vi "Emulator_VI_template.vi"() -> ()   [LabVIEW 2020]
uses:
  <vilib>/Instr/_visa.llb/VISA Configure Serial Port (Instr).vi
panel:
  in  "Start":bool
  in  "Stop":bool
  in  "Serial port configuration":T1={"Baud rate"=0, "Data bits"=5, "Parity"=enum."None", "Stop bits"=0, "Flow control"=0} {"Flow control" items=["None"=0, "XON/XOFF"=1, "RTS/CTS"=2, "DTR/DSR"=4]; "Stop bits" items=["1.0"=10, "1.5"=15, "2.0"=20]; "Data bits" min=5 max=8 step=1; "Baud rate" items=["9600"=9600, "19200"=19200, "38400"=38400, "57600"=57600, "115200"=115200]}
  in  "Port":refnum<visa-resource-name>
  # "Project name:  Emulator_VI_template.vi \nDescription:     Template VI for emulation interface communicating with external target through UART port\nVersion:           01.00\nRevision:          00\nLast modified : MM/DD/YYYY"
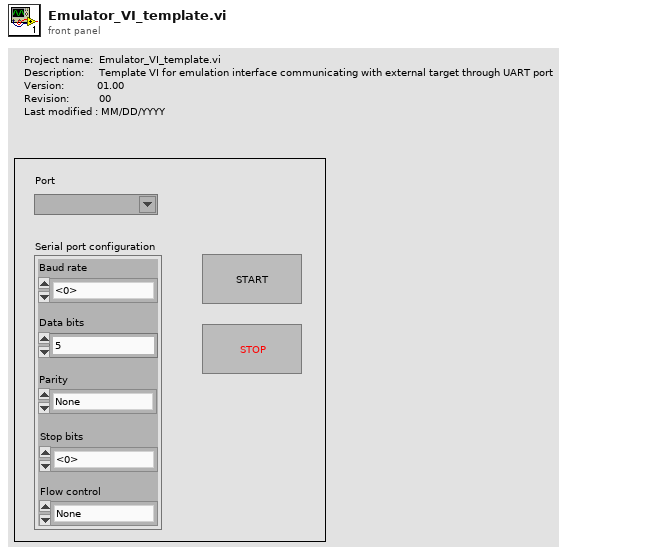
[diagram p1: front panel]
types:
  T1 = cluster{"Baud rate":u32, "Data bits":u16, "Parity":enum16{"None", "Odd", "Even", "Mark", "Space"}, "Stop bits":u16, "Flow control":u16}
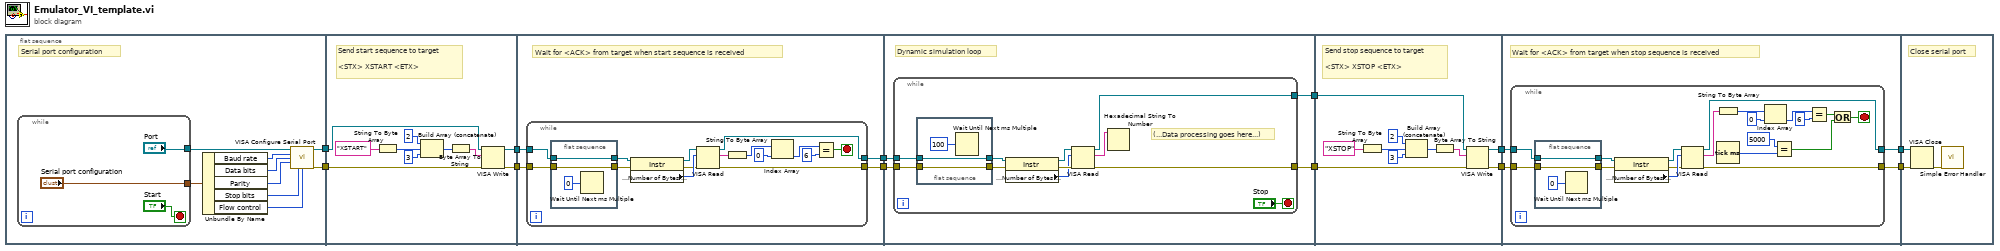
[diagram p0: block diagram]
diagram:
  n1 = flat-sequence {
    tunnel: [w14] -> w12
    tunnel: [w13] -> w11
    tunnel: w12 -> [w34]
    tunnel: w11 -> [w33]
    tunnel: [w26] -> w10
    tunnel: [w25] -> w9
    tunnel: w10 -> [w38]
    tunnel: w9 -> [w37]
    tunnel: [w36] -> w8
    tunnel: [w35] -> w7
    tunnel: w8 -> [w60]
    tunnel: w7 -> [w59]
    tunnel: [w58] -> w4
    tunnel: [w57] -> w3
    tunnel: [w78] -> w6
    tunnel: [w77] -> w5
    tunnel: w4 -> [w76]
    tunnel: w3 -> [w75]
    tunnel: w6 -> [w88]
    tunnel: w5 -> [w87]
    tunnel: [w86] -> w2
    tunnel: [w85] -> w1
    tunnel: w2 -> [w112]
    tunnel: w1 -> [w111]
    frame #0 {
      # "Serial port configuration"
      n2 = while {
        tunnel: ["Port"] -> w15
        tunnel: ["Serial port configuration"] -> w16
        stop <- "Start" stop-if-true
      }
      n3 = Unbundle By Name(w16) -> ("Baud rate"=w17:u32, "Data bits"=w18:u16, "Parity"=w19:enum16{"None", "Odd", "Even", "Mark", "Space"}, "Stop bits"=w20:u16, "Flow control"=w21:u16)
      n4 = call-poly "VISA Configure Serial Port"("VISA resource name"=w15, "baud rate (9600)"=w17, "data bits (8)"=w18, "parity (0:none)"=w19, "stop bits (10: 1 bit)"=w20, "flow control (0:none)"=w21) -> ("VISA resource name out"=w13:refnum<visa-resource-name>, "error out"=w14:errorcluster)  [unwired: 8 in]
    }
    frame #1 {
      # "Send start sequence to target \n\n<STX> XSTART <ETX>"
      n5 = String To Byte Array(string="XSTART") -> (unsigned byte array=w32:u8[])
      n6 = Build Array (concatenate)(u8 2, w32, u8 3) -> (w31:u8[])
      n7 = Byte Array To String(unsigned byte array=w31) -> (string=w27:string)
      n8 = VISA Write(VISA resource name=w33, write buffer=w27, error in (no error)=w34) -> (VISA resource name out=w26:refnum<visa-resource-name>, error out=w25:errorcluster)  [unwired: 1 out]
    }
    frame #2 {
      # "Wait for <ACK> from target when start sequence is received"
      n9 = while {
        tunnel: w38 -> [w48]
        tunnel: w37 -> [w47]
        tunnel: [w40] -> w36
        tunnel: [w39] -> w35
        stop <- w41 stop-if-true
        n10 = flat-sequence {
          tunnel: w48 -> [w56]
          tunnel: w47 -> [w55]
          tunnel: [w56] -> w52
          tunnel: [w55] -> w53
          frame #0 {
            n11 = Wait Until Next ms Multiple(millisecond multiple=u32 0) -> ()  [unwired: 1 out]
          }
        }
        n12 = property class="Instr"(reference=w52, error in=w53) -> (reference out=w49:refnum<visa-resource-name>, error out=w50:errorcluster, "Serial Settings:Number of Bytes at Serial Port"=w51:u32)
        n13 = VISA Read(VISA resource name=w49, byte count=w51, error in (no error)=w50) -> (VISA resource name out=w40:refnum<visa-resource-name>, read buffer=w42:string, error out=w39:errorcluster)  [unwired: 1 out]
        n14 = String To Byte Array(string=w42) -> (unsigned byte array=w46:u8[])
        n15 = Index Array(array=w46, index=0) -> (element=w44:u8)
        n16 = Equal?(x=w44, y=u8 6) -> (x = y?=w41:bool)
      }
    }
    frame #3 {
      # "Dynamic simulation loop"
      n17 = while {
        tunnel: w60 -> [w64]
        tunnel: w59 -> [w63]
        tunnel: [w70] -> w57
        tunnel: [w69] -> w58
        stop <- "Stop" stop-if-true
        # "(...Data processing goes here...)"
        n18 = flat-sequence {
          tunnel: w64 -> [w73]
          tunnel: w63 -> [w72]
          tunnel: [w73] -> w62
          tunnel: [w72] -> w61
          frame #0 {
            n19 = Wait Until Next ms Multiple(millisecond multiple=u32 100) -> ()  [unwired: 1 out]
          }
        }
        n20 = property class="Instr"(reference=w62, error in=w61) -> (reference out=w67:refnum<visa-resource-name>, error out=w66:errorcluster, "Serial Settings:Number of Bytes at Serial Port"=w65:u32)
        n21 = VISA Read(VISA resource name=w67, byte count=w65, error in (no error)=w66) -> (VISA resource name out=w69:refnum<visa-resource-name>, read buffer=w68:string, error out=w70:errorcluster)  [unwired: 1 out]
        n22 = Hexadecimal String To Number(string=w68) -> ()  [unwired: 2 in, 2 out]
      }
    }
    frame #4 {
      # "Send stop sequence to target \n\n<STX> XSTOP <ETX>"
      n23 = String To Byte Array(string="XSTOP") -> (unsigned byte array=w84:u8[])
      n24 = Build Array (concatenate)(u8 2, w84, u8 3) -> (w83:u8[])
      n25 = Byte Array To String(unsigned byte array=w83) -> (string=w82:string)
      n26 = VISA Write(VISA resource name=w76, write buffer=w82, error in (no error)=w75) -> (VISA resource name out=w78:refnum<visa-resource-name>, error out=w77:errorcluster)  [unwired: 1 out]
    }
    frame #5 {
      # "Wait for <ACK> from target when stop sequence is received"
      n27 = while {
        tunnel: [w97] -> w86
        tunnel: [w96] -> w85
        tunnel: w87 -> [w95]
        tunnel: w88 -> [w94]
        stop <- w89 stop-if-true
        n28 = flat-sequence {
          tunnel: [w108] -> w106
          tunnel: [w109] -> w107
          tunnel: w95 -> [w109]
          tunnel: w94 -> [w108]
          frame #0 {
            n29 = Wait Until Next ms Multiple(millisecond multiple=u32 0) -> ()  [unwired: 1 out]
          }
        }
        n30 = property class="Instr"(reference=w106, error in=w107) -> (reference out=w103:refnum<visa-resource-name>, error out=w104:errorcluster, "Serial Settings:Number of Bytes at Serial Port"=w105:u32)
        n31 = VISA Read(VISA resource name=w103, byte count=w105, error in (no error)=w104) -> (VISA resource name out=w97:refnum<visa-resource-name>, read buffer=w98:string, error out=w96:errorcluster)  [unwired: 1 out]
        n32 = String To Byte Array(string=w98) -> (unsigned byte array=w102:u8[])
        n33 = Tick Count (ms)() -> (millisecond timer value=w93:u32)
        n34 = Index Array(array=w102, index=0) -> (element=w100:u8)
        n35 = Equal?(x=u32 5000, y=w93) -> (x = y?=w91:bool)
        n36 = Equal?(x=w100, y=u8 6) -> (x = y?=w90:bool)
        n37 = Or(x=w90, y=w91) -> (x .or. y?=w89:bool)
      }
    }
    frame #6 {
      # "Close serial port"
      n38 = VISA Close(VISA resource name=w112, error in (no error)=w111) -> (error out=w113:errorcluster)
      n39 = call <vilib>:"Simple Error Handler.vi"("error in (no error)"=w113) -> ()  [unwired: 4 in, 5 out]
    }
  }
